vi "Set Number of Test Methods.vi"(8 "error in (no error)":errorcluster, 10 "Method Count":u32, 11 "Result Table.lvclass":refnum<class "Result Table.lvclass">) -> (0 "error out":errorcluster, 3 "Result Table":refnum<class "Result Table.lvclass">)   [LabVIEW 2020, in "Result Table.lvclass"]
uses:
  Result Table.lvclass
  Private/TypeDefs/Table Columns.ctl
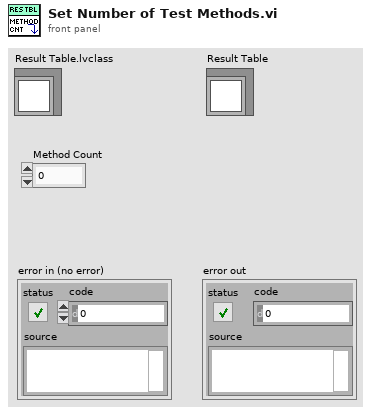
[diagram p1: front panel]
types:
  T1 = typedef "Result Table.lvclass/Table Columns.ctl" = u16
  T2 = typedef "Results.ctl" = cluster{"Method Count":u32, "Executed Methods":u32, "Passed Methods":u32, "Failed Methods":u32, "Method Errors":u32, "Skipped Method":u32}
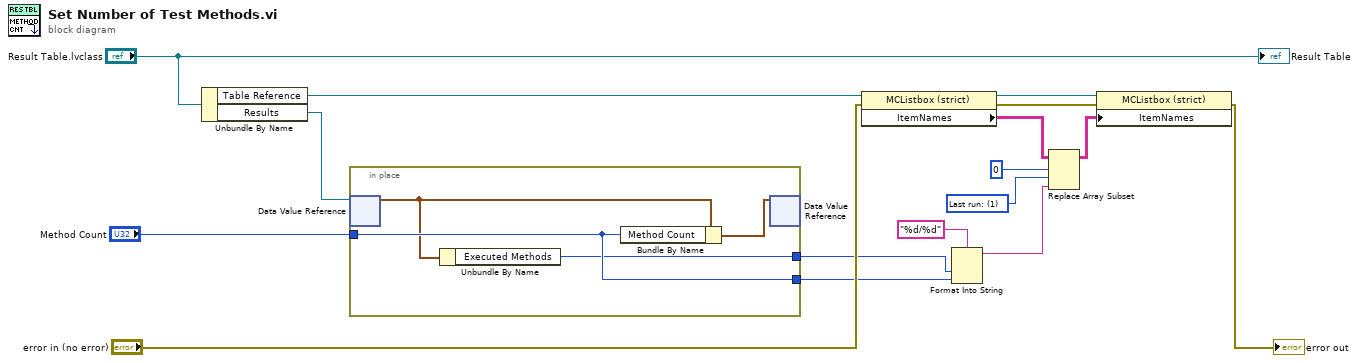
[diagram p0: block diagram]
diagram:
  w10 = T1 1 items=["Last run:"=1, "Passed:"=3, "Failed:"=5, "Errors:"=7, "Skipped"=9] ("Table Columns")
  n1 = Unbundle By Name("Result Table.lvclass") -> ("Table Reference"=w5:refnum<vi>, "Results"=w12:refnum<data-value>)
  n2 = in-place {
    in-place-border: "Method Count" -> [w19]
    in-place-border: [w19] -> w2
    in-place-border: [w17] -> w3
    n3 = in-place-dvr #1(w12) -> (w18:T2)  [unwired: 1 out]
    n4 = Unbundle By Name(w18) -> ("Executed Methods"=w17:u32)
    n5 = Bundle By Name(cluster=w18, "Method Count"=w19) -> (w20:T2)
    n6 = in-place-dvr #1(w20) -> ()  [unwired: 2 out]
  }
  n7 = property class="MCListbox (strict)"(reference=w5, error in="error in (no error)") -> (reference out=w6:refnum<vi>, error out=w7:errorcluster, "ItemNames"=w11:string[][])
  n8 = Format Into String(format string="%d/%d", w3, w2) -> (resulting string=w1:string)  [unwired: 2 in, 1 out]
  n9 = Replace Array Subset(array=w11, new element=w1, index (row)=0 ("disabled index (row)"), index (col)=w10) -> (w8:string[][])
  n10 = property class="MCListbox (strict)"(reference=w6, error in=w7, "ItemNames"=w8) -> (error out=→"error out":errorcluster)  [unwired: 1 out]
  "Result Table" <- "Result Table.lvclass"
